vi "Set_output_channel_group.vi"(8 "error in (no error)":errorcluster, 9 "Group_output":T1, 10 "Channel_output":dbl[](array[numeric]), 11 "Toolbox in":refnum<class "Toolbox.lvclass">) -> (0 "error out":errorcluster, 3 "Toolbox out":refnum<class "Toolbox.lvclass">)   [LabVIEW 2014, in "Driver_interaction.lvlib" / "Toolbox.lvclass"]
uses:
  Toolbox.lvclass
  Controls/Group_output.ctl
  Controls/Group_selector.ctl
  _Driver_interaction/_Driver_interaction.lvclass/_Driver_interaction.ctl
  Toolbox.lvclass/Toolbox.ctl
  _Driver_interaction/_Driver_interaction.lvclass
  Vendor/lib 2p0/FTS 2p0.lvlib
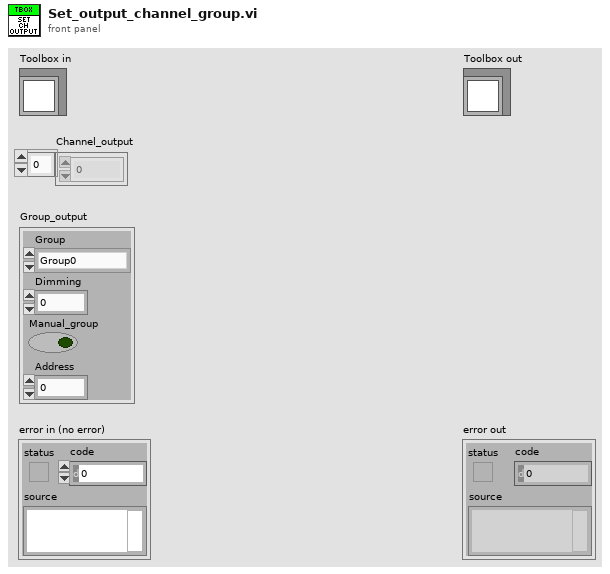
[diagram p1: front panel]
types:
  T1 = typedef "Driver_interaction.lvlib/Toolbox.lvclass/Group_output.ctl" = cluster{"Group":T2, "Dimming":i32, "Manual_group":bool, "Address":i32}
  T2 = typedef "Driver_interaction.lvlib/Toolbox.lvclass/Group_selector.ctl" = enum16{"Group0", "Group1", "Group2", "Group3", "Group4", "Group5", "Group6", "Group7", "Group8", "Group9", "Group10", "Group11", "Group12", "Group13", "Group14", "Group15", "All Groups"}
  T3 = typedef "Driver_interaction.lvlib/_Driver_interaction.lvclass/Interface_type.ctl" = string
  T4 = typedef "Driver_interaction.lvlib/Toolbox.lvclass/Toolbox_session.ctl" = cluster{"client handle":T5, "URL out":string, "universe_id":i32, "devices_id":i32[]}
  T5 = typedef "LabVIEWHTTPClient.lvlib/ClientHandle.ctl" = refnum<k1>
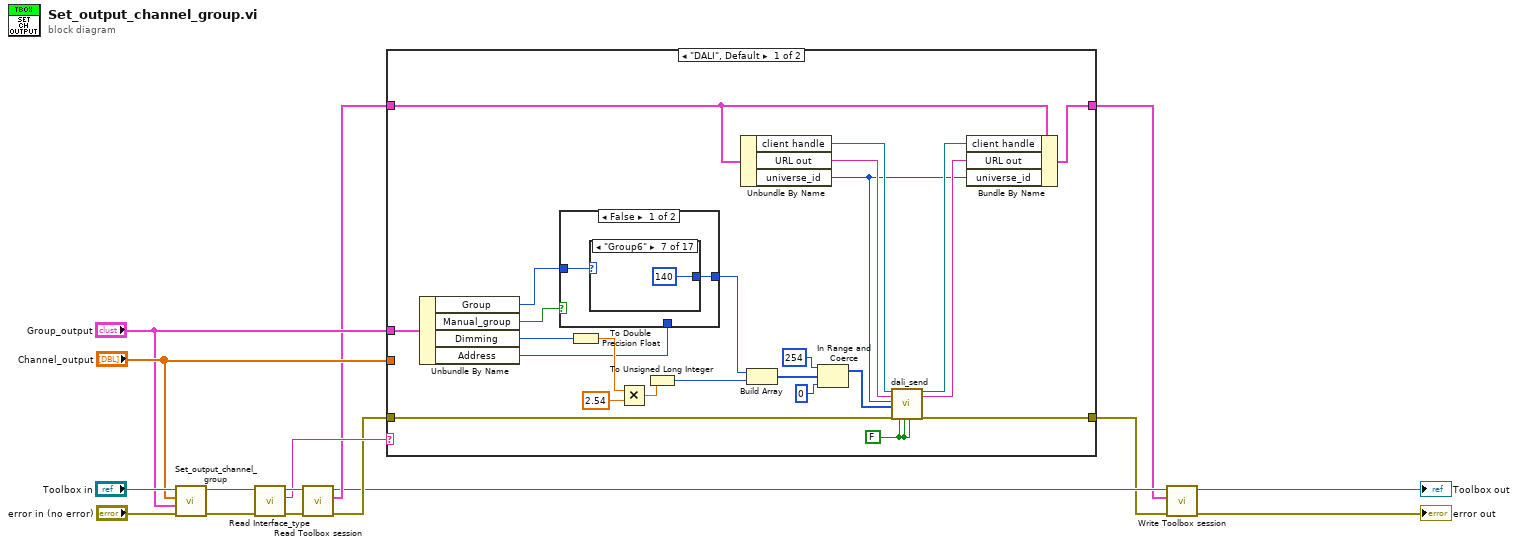
[diagram p0: block diagram]
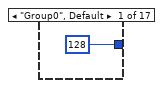
[diagram p2: hidden frame]
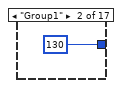
[diagram p3: hidden frame]
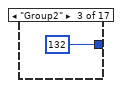
[diagram p4: hidden frame]
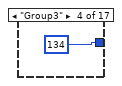
[diagram p5: hidden frame]
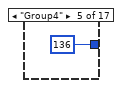
[diagram p6: hidden frame]
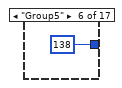
[diagram p7: hidden frame]
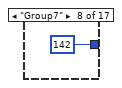
[diagram p8: hidden frame]
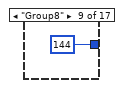
[diagram p9: hidden frame]
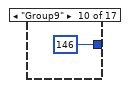
[diagram p10: hidden frame]
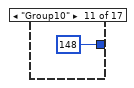
[diagram p11: hidden frame]
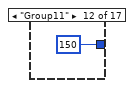
[diagram p12: hidden frame]
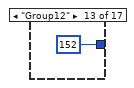
[diagram p13: hidden frame]
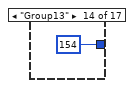
[diagram p14: hidden frame]
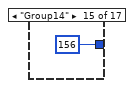
[diagram p15: hidden frame]
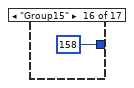
[diagram p16: hidden frame]
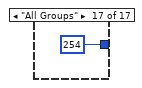
[diagram p17: hidden frame]
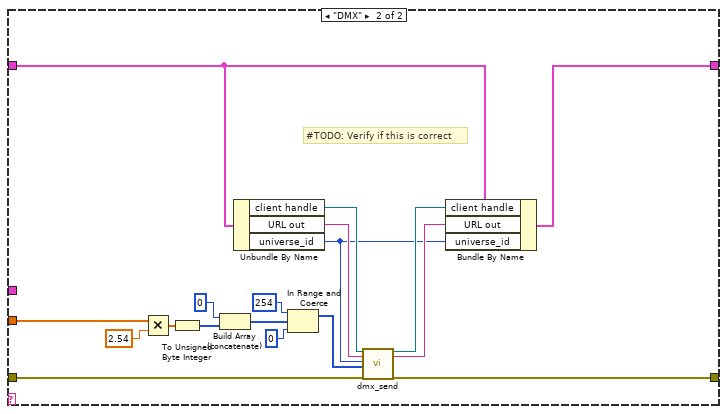
[diagram p19: hidden frame]
diagram:
  n1 = call-parent "Set_output_channel_group.vi"("error in (no error)"="error in (no error)", "Group_output"="Group_output", "Channel_output"="Channel_output", "_Driver_interaction in"="Toolbox in") -> ("error out"=w14:errorcluster, "_Driver_interaction out"=w13:refnum<class "Toolbox.lvclass">)  [unwired: 6 in]
  n2 = call "Read Interface_type.vi"("error in (no error)"=w14, "_Driver_interaction in"=w13) -> ("error out"=w9:errorcluster, "Interface_type"=w8:T3, "_Driver_interaction out"=w10:refnum<class "Toolbox.lvclass">)  [unwired: 7 in]
  n3 = call "Read Toolbox session.vi"("error in (no error)"=w9, "Toolbox in"=w10) -> ("error out"=w6:errorcluster, "Toolbox session"=w7:T4, "Toolbox out"=w5:refnum<class "Toolbox.lvclass">)  [unwired: 7 in]
  n4 = case shown="\"DALI\", Default" w8 {
    tunnel: w7 -> [w21 w67]
    tunnel: w6 -> [w40 w71]
    tunnel: [w17 w63] -> w4
    tunnel: "Channel_output" -> [_ w62]
    tunnel: [w39 w61] -> w3
    tunnel: "Group_output" -> [w30 _]
    frame "DALI", Default {
      w38 = FALSE ("params.expect_answer")
      n5 = Unbundle By Name(w30) -> ("Group"=w25:T2, "Manual_group"=w26:bool, "Dimming"=w29:i32, "Address"=w27:i32)
      n6 = case shown="False" w26 {
        tunnel: w25 -> [w42 _]
        tunnel: [w41 w60] -> w34
        tunnel: w27 -> [_ w60]
        frame False {
          n7 = case shown="\"Group6\"" w42 {
            tunnel: [128 130 132 134 136 138 140 142 144 146 148 150 152 154 156 158 254] -> w41
            frame "Group0", Default {
            }
            frame "Group1" {
            }
            frame "Group2" {
            }
            frame "Group3" {
            }
            frame "Group4" {
            }
            frame "Group5" {
            }
            frame "Group6" {
            }
            frame "Group7" {
            }
            frame "Group8" {
            }
            frame "Group9" {
            }
            frame "Group10" {
            }
            frame "Group11" {
            }
            frame "Group12" {
            }
            frame "Group13" {
            }
            frame "Group14" {
            }
            frame "Group15" {
            }
            frame "All Groups" {
            }
          }
        }
        frame True {
        }
      }
      n8 = To Double Precision Float(number=w29) -> (double precision float=w28:dbl)
      n9 = Multiply(x=w28, y=2.54) -> (x*y=w32:dbl)
      n10 = To Unsigned Long Integer(number=w32) -> (unsigned 32bit integer=w31:u32)
      n11 = Unbundle By Name(w21) -> ("client handle"=w23:T5, "URL out"=w22:string, "universe_id"=w18:i32)
      n12 = Build Array(w34, w31) -> (w35:u32[])
      n13 = In Range and Coerce(upper limit=u8 254, x=w35, lower limit=u8 0) -> (coerced(x)=w24:u32[])  [unwired: 1 out]
      n14 = call "dali_send.vi"("client handle"=w23, "URL"=w22, "params.universe_id"=w18, "params.bytes"=w24, "error in (no error)"=w40, "params.expect_answer"=w38, "params.send_twice"=w38, "params.internal_addressing"=w38) -> ("client handle out"=w20:T5, "URL out"=w19:string, "error out"=w39:errorcluster)  [unwired: 8 in, 1 out]
      n15 = Bundle By Name(cluster=w21, "client handle"=w20, "URL out"=w19, "universe_id"=w18) -> (w17:T4)
    }
    frame "DMX" {
      # "#TODO: Verify if this is correct"
      n16 = Multiply(x=w62, y=2.54) -> (x*y=w74:dbl[])
      n17 = To Unsigned Byte Integer(number=w74) -> (unsigned 8bit integer=w75:u8[])
      n18 = Build Array (concatenate)(u8 0, w75) -> (w76:u8[])
      n19 = Unbundle By Name(w67) -> ("client handle"=w70:T5, "URL out"=w69:string, "universe_id"=w64:i32)
      n20 = In Range and Coerce(upper limit=u8 254, x=w76, lower limit=u8 0) -> (coerced(x)=w68:u8[])  [unwired: 1 out]
      n21 = call "dmx_send.vi"("client handle"=w70, "URL"=w69, "params.universe_id"=w64, "params.bytes"=w68, "error in (no error)"=w71) -> ("client handle out"=w66:T5, "URL out"=w65:string, "error out"=w61:errorcluster)  [unwired: 11 in, 1 out]
      n22 = Bundle By Name(cluster=w67, "client handle"=w66, "URL out"=w65, "universe_id"=w64) -> (w63:T4)
    }
  }
  n23 = call "Write Toolbox session.vi"("error in (no error)"=w3, "Toolbox session"=w4, "Toolbox in"=w5) -> ("error out"=→"error out":errorcluster, "Toolbox out"=→"Toolbox out":refnum<class "Toolbox.lvclass">)  [unwired: 7 in]
